vi "BMark_Get VIs in Project.vi"(8 "Error In":errorcluster, 11 "project":refnum<vi>) -> (0 "Error Out":errorcluster, 2 "Array of VIs":T1[](array[typedef]), 3 "project out":refnum<vi>)   [LabVIEW 2018, in "Bookmark Manager.lvlib"]
uses:
  Bookmark Manager.lvlib
  Controls/BMark_VI_Identifier.ctl
  <vilib>/addons/analyzer/_analyzerctrls.llb/VIAnCtl Analysis App Info.ctl
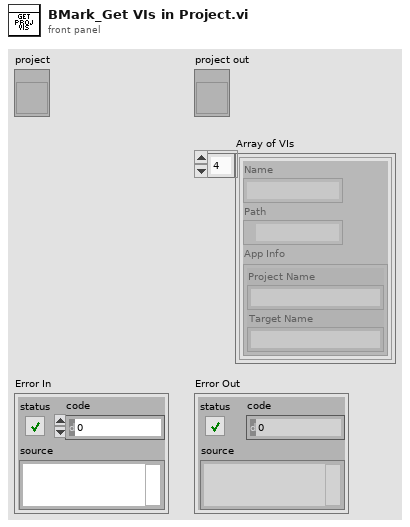
[diagram p1: front panel]
types:
  T1 = typedef "Bookmark Manager.lvlib/BMark_VI_Identifier.ctl" = cluster{"Name":string, "Path":path, "App Info":T2}
  T2 = typedef "VIAnCtl Analysis App Info.ctl" = cluster{"Project Name":string, "Target Name":string}
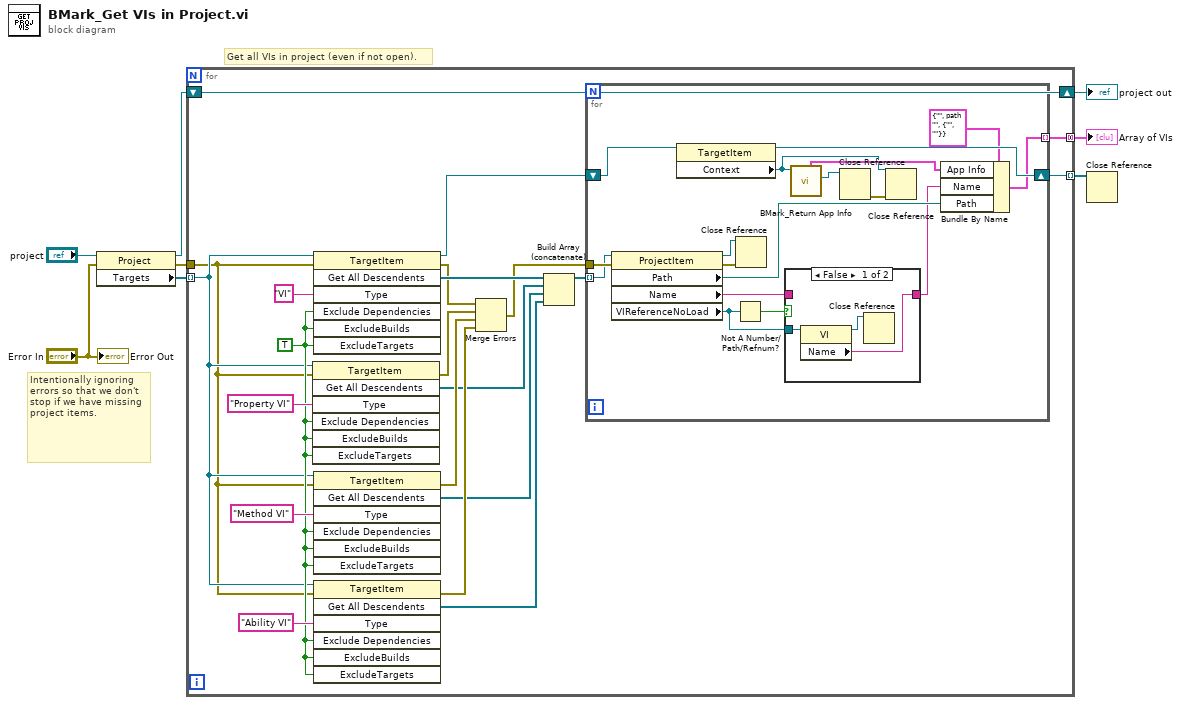
[diagram p0: block diagram]
diagram:
  # "Intentionally ignoring errors so that we don't stop if we have missing project items."
  # "Get all VIs in project (even if not open)."
  n1 = property class="Project"(reference="project", error in="Error In") -> (reference out=w2:refnum<vi>, error out=w6:errorcluster, "Targets"=w8:refnum<vi>[])
  n2 = for {
    tunnel: w8 -> [w17] mode=indexing
    tunnel: [w27] -> w5 mode=indexing
    tunnel: [w26] -> w4 mode=concatenating
    tunnel: w6 -> [w16]
    shift-right: [w25] -> w1
    shift-left: w2 -> [w25]
    w18 = TRUE ("ExcludeDependencies")
    n3 = invoke class="TargetItem" method="Get All Descendents"(reference=w17, error in=w16, "Type"="Property VI", "Exclude Dependencies"=w18, "ExcludeBuilds"=w18, "ExcludeTargets"=w18) -> (error out=w15:errorcluster, "All Descendents"=w11:refnum<vi>[])  [unwired: 1 in, 5 out]
    n4 = invoke class="TargetItem" method="Get All Descendents"(reference=w17, error in=w16, "Type"="VI", "Exclude Dependencies"=w18, "ExcludeBuilds"=w18, "ExcludeTargets"=w18) -> (reference out=w28:refnum<vi>, error out=w23:errorcluster, "All Descendents"=w29:refnum<vi>[])  [unwired: 1 in, 4 out]
    n5 = invoke class="TargetItem" method="Get All Descendents"(reference=w17, error in=w16, "Type"="Method VI", "Exclude Dependencies"=w18, "ExcludeBuilds"=w18, "ExcludeTargets"=w18) -> (error out=w14:errorcluster, "All Descendents"=w10:refnum<vi>[])  [unwired: 1 in, 5 out]
    n6 = invoke class="TargetItem" method="Get All Descendents"(reference=w17, error in=w16, "Type"="Ability VI", "Exclude Dependencies"=w18, "ExcludeBuilds"=w18, "ExcludeTargets"=w18) -> (error out=w13:errorcluster, "All Descendents"=w9:refnum<vi>[])  [unwired: 1 in, 5 out]
    n7 = Merge Errors(w23, w15, w14, w13) -> (w22:errorcluster)
    n8 = Build Array (concatenate)(w29, w11, w10, w9) -> (w12:refnum<vi>[])
    n9 = for {
      tunnel: w12 -> [w32] mode=indexing
      shift-right: [w43] -> w27
      shift-left: w28 -> [w30]
      tunnel: [w40] -> w26 mode=indexing
      tunnel: w22 -> [w46]
      n10 = property class="ProjectItem"(reference=w32, error in=w46) -> (reference out=w44:refnum<vi>, error out=w45:errorcluster, "Path"=w41:path, "Name"=w38:string, "VIReferenceNoLoad"=w31:refnum<vi>)
      n11 = property class="TargetItem"(reference=w30) -> (reference out=w43:refnum<vi>, "Context"=w33:refnum<vi>)  [unwired: 1 in, 1 out]
      n12 = Not A Number/Path/Refnum?(number/path/refnum=w31) -> (NaN/Path/Refnum?=w39:bool)
      n13 = Close Reference(reference=w44, error in (no error)=w45) -> ()  [unwired: 1 out]
      n14 = case shown="False" w39 {
        tunnel: w38 -> [_ w50]
        tunnel: [w48 w50] -> w37
        tunnel: w31 -> [w49 _]
        frame False {
          n15 = property class="VI"(reference=w49) -> (reference out=w47:refnum<vi>, "Name"=w48:string)  [unwired: 1 in, 1 out]
          n16 = Close Reference(reference=w47) -> ()  [unwired: 1 in, 1 out]
        }
        frame True {
        }
      }
      n17 = call "BMark_Return App Info.vi"("App Refnum in"=w33) -> ("App Refnum for Opening VI"=w35:refnum<vi>, "App Info"=w36:T2)  [unwired: 8 in, 1 out]
      n18 = Close Reference(reference=w35) -> (error out=w34:errorcluster)  [unwired: 1 in]
      n19 = Close Reference(reference=w33, error in (no error)=w34) -> ()  [unwired: 1 out]
      n20 = Bundle By Name(cluster=T1 {"Name"="", "Path"=path "", "App Info"={"Project Name"="", "Target Name"=""}}, "App Info"=w36, "Name"=w37, "Path"=w41) -> (w40:T1)
    }
  }
  "Array of VIs" <- w4
  "project out" <- w1
  n21 = Close Reference(reference=w5) -> ()  [unwired: 1 in, 1 out]
  "Error Out" <- "Error In"
